vi "findE_B.vi"(4 "lastR":dbl, 5 "time":dbl[](array[numeric]), 6 "lastE":dbl, 7 "Ve":dbl[](array[numeric])) -> (0 "VE_B":dbl[](array[numeric]), 1 "VE_E":dbl[](array[numeric]), 2 "time_B":dbl[](array[numeric]), 3 "time_E":dbl[](array[numeric]))   [LabVIEW 2011]
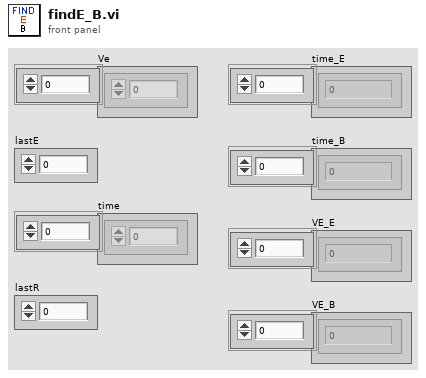
[diagram p1: front panel]
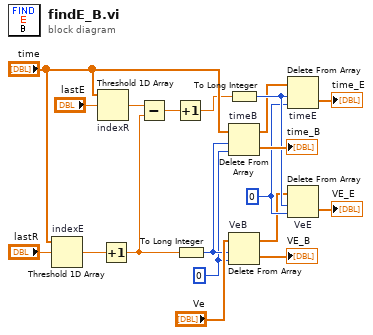
[diagram p0: block diagram]
diagram:
  w4 = 0 ("index")
  w1 = 0 ("index")
  n1 = Threshold 1D Array "indexE"(2:"lastR", 3:"time") -> (0:w6:dbl)  [unwired: 1 in]
  n2 = Threshold 1D Array "indexR"(2:"lastE", 3:"time") -> (0:w5:dbl)  [unwired: 1 in]
  n3 = Increment(x=w6) -> (x+1=w10:dbl)
  n4 = Subtract(x=w5, y=w10) -> (x-y=w7:dbl)
  n5 = Increment(x=w7) -> (x+1=w11:dbl)
  n6 = To Long Integer(number=w10) -> (32bit integer=w9:i32)
  n7 = To Long Integer(number=w11) -> (32bit integer=w8:i32)
  n8 = Delete From Array "timeB"(array="time", length=w9, index=w1) -> (deleted portion=→"time_B":dbl[], array with subset deleted=w2:dbl[])
  n9 = Delete From Array "VeB"(array="Ve", length=w9, index=w1) -> (deleted portion=→"VE_B":dbl[], array with subset deleted=w3:dbl[])
  n10 = Delete From Array "timeE"(array=w2, length=w8, index=w4) -> (deleted portion=→"time_E":dbl[])  [unwired: 1 out]
  n11 = Delete From Array "VeE"(array=w3, length=w8, index=w4) -> (deleted portion=→"VE_E":dbl[])  [unwired: 1 out]
